vi "log analysis_gps.vi"() -> ()   [LabVIEW 2019] (continued)
0.4458,0.2943,0.5547,0.1143,0.0925,0.0773,0.0983,0.1035,4.8018,0f000001,0*da40ff02\n\t", "INSPVAXA,USB3,0,50.0,FINESTEERING,2107,282792.500,02000000,471d,15824;INS_ALIGNMENT_COMPLETE,INS_RTKFIXED,37.37073031281,126.72411271384,9.9474,22.3000,0.1838,-0.2244,-0.0278,-0.319663676,-2.204085935,299.407243986,0.4460,0.2943,0.5548,0.1143,0.0925,0.0773,0.0983,0.1036,4.8027,0f000001,0*a7b7d02c\n\t", "INSPVAXA,USB3,0,50.0,FINESTEERING,2107,282793.000,02000000,471d,15824;INS_ALIGNMENT_COMPLETE,INS_RTKFIXED,37.37073105512,126.72411141845,9.9418,22.3000,0.2101,-0.2661,-0.0283,-0.304105156,-2.230574791,299.428124027,0.4460,0.2943,0.5548,0.1143,0.0925,0.0773,0.0983,0.1036,4.8027,0f000001,0*32017f41\n\t", "INSPVAXA,USB3,0,48.5,FINESTEERING,2107,282793.500,02000000,471d,15824;INS_ALIGNMENT_COMPLETE,INS_RTKFIXED,37.37073179967,126.72411009506,9.9373,22.3000,0.1839,-0.2284,-0.0293,-0.261169015,-2.357198246,299.469051976,0.4470,0.2945,0.5553,0.1144,0.0927,0.0774,0.0983,0.1036,4.8035,0f000001,0*5198649b\n\t", "INSPVAXA,USB3,0,48.5,FINESTEERING,2107,282794.000,02000000,471d,15824;INS_ALIGNMENT_COMPLETE,INS_RTKFIXED,37.37073258034,126.72410870830,9.9322,22.3000,0.1804,-0.2290,-0.0311,-0.237665421,-2.328772316,299.577236299,0.4470,0.2945,0.5553,0.1144,0.0927,0.0774,0.0983,0.1036,4.8035,0f000001,0*00fdb5a8\n\t", "INSPVAXA,USB3,0,50.0,FINESTEERING,2107,282794.500,02000000,471d,15824;INS_ALIGNMENT_COMPLETE,INS_RTKFIXED,37.37073330075,126.72410740472,9.9287,22.3000,0.1893,-0.2427,-0.0278,-0.202786531,-2.243456476,299.635927133,0.4467,0.2943,0.5552,0.1145,0.0925,0.0773,0.0983,0.1036,4.8037,0f000001,0*5cb0ba92\n\t", "INSPVAXA,USB3,0,50.0,FINESTEERING,2107,282795.000,02000000,471d,15824;INS_ALIGNMENT_COMPLETE,INS_RTKFIXED,37.37073403278,126.72410609803,9.9257,22.3000,0.2016,-0.2553,-0.0322,-0.209242337,-1.998269327,299.675209205,0.4467,0.2943,0.5552,0.1145,0.0925,0.0773,0.0983,0.1036,4.8037,0f000001,0*b5d55d6c\n\t", "INSPVAXA,USB3,0,47.5,FINESTEERING,2107,282795.500,02000000,471d,15824;INS_ALIGNMENT_COMPLETE,INS_RTKFIXED,37.37073477439,126.72410478765,9.9228,22.3000,0.1988,-0.2433,-0.0255,-0.169516872,-1.839910246,299.717118650,0.4468,0.2942,0.5552,0.1144,0.0925,0.0773,0.0984,0.1036,4.8041,0f000001,0*ac4c0833\n\t", "DUALANTENNAHEADINGA,USB3,0,47.5,FINESTEERING,2107,282796.000,02000000,d426,15824;INSUFFICIENT_OBS,NONE,-1.000000000,0.000000000,0.000000000,0.0,0.000000000,0.000000000,\"631T\",16,2,2,2,04,00,20,00*03fa76b0\n\t", "INSPVAXA,USB3,0,49.5,FINESTEERING,2107,282796.500,02000000,471d,15824;INS_ALIGNMENT_COMPLETE,INS_RTKFIXED,37.37073628296,126.72410213089,9.9158,22.3000,0.1865,-0.2481,-0.0343,-0.084207342,-1.811662938,299.819471466,0.4465,0.2941,0.5548,0.1145,0.0924,0.0773,0.0984,0.1036,4.8046,0f000001,0*5f5dfc2c\n\t", "DUALANTENNAHEADINGA,USB3,0,49.5,FINESTEERING,2107,282797.000,02000000,d426,15824;INSUFFICIENT_OBS,NONE,-1.000000000,0.000000000,0.000000000,0.0,0.000000000,0.000000000,\"631T\",11,2,2,2,04,00,20,00*3233b119\n\t", "INSPVAXA,USB3,0,51.0,FINESTEERING,2107,282797.500,02000000,471d,15824;INS_ALIGNMENT_COMPLETE,INS_RTKFIXED,37.37073777614,126.72409945855,9.9099,22.3000,0.1844,-0.2371,-0.0242,-0.262384878,-2.080175298,299.815880388,0.4468,0.2941,0.5547,0.1144,0.0924,0.0773,0.0984,0.1036,4.8050,0f000001,0*8c5fb6f4\n\t", "DUALANTENNAHEADINGA,USB3,0,51.0,FINESTEERING,2107,282798.000,02000000,d426,15824;INSUFFICIENT_OBS,NONE,-1.000000000,0.000000000,0.000000000,0.0,0.000000000,0.000000000,\"631T\",13,2,2,2,04,00,20,00*54bdf9a5\n\t", "DUALANTENNAHEADINGA,USB3,0,48.5,FINESTEERING,2107,282798.500,02000000,d426,15824;INSUFFICIENT_OBS,NONE,-1.000000000,0.000000000,0.000000000,0.0,0.000000000,0.000000000,\"631T\",13,2,2,2,04,00,20,00*f78b4211\n\t", "INSPVAXA,USB3,0,48.5,FINESTEERING,2107,282799.000,02000000,471d,15824;INS_ALIGNMENT_COMPLETE,INS_RTKFIXED,37.37074001096,126.72409550695,9.9018,22.3000,0.1871,-0.2390,-0.0286,-0.222837018,-2.091989069,299.851600763,0.4467,0.2941,0.5546,0.1145,0.0924,0.0773,0.0984,0.1036,4.8055,0f000001,0*154119ed\n\t", "INSPVAXA,USB3,0,48.0,FINESTEERING,2107,282799.500,02000000,471d,15824;INS_ALIGNMENT_COMPLETE,INS_RTKFIXED,37.37074075005,126.72409418540,9.8978,22.3000,0.1813,-0.2293,-0.0193,-0.296668492,-2.062854317,299.895574277,0.4469,0.2941,0.5547,0.1144,0.0924,0.0773,0.0985,0.1036,4.8059,0f000001,0*557f2fd1\n\t", "INSPVAXA,USB3,0,48.0,FINESTEERING,2107,282800.000,02000000,471d,15824;INS_ALIGNMENT_COMPLETE,INS_RTKFIXED,37.37074149494,126.72409286106,9.8944,22.3000,0.1833,-0.2479,-0.0244,-0.375636327,-2.245041894,299.896302450,0.4469,0.2941,0.5547,0.1144,0.0924,0.0773,0.0985,0.1036,4.8059,0f000001,0*618fc424\n\t", "INSPVAXA,USB3,0,50.5,FINESTEERING,2107,282800.500,02000000,471d,15824;INS_ALIGNMENT_COMPLETE,INS_RTKFIXED,37.37074223493,126.72409154227,9.8930,22.3000,0.1953,-0.2548,-0.0229,-0.359173553,-2.315682427,299.885169095,0.4472,0.2942,0.5548,0.1143,0.0924,0.0774,0.0985,0.1036,4.8064,0f000001,0*7582bc0e\n\t", "INSPVAXA,USB3,0,50.5,FINESTEERING,2107,282801.000,02000000,471d,15824;INS_ALIGNMENT_COMPLETE,INS_RTKFIXED,37.37074297365,126.72409022766,9.8906,22.3000,0.1848,-0.2408,-0.0220,-0.434084237,-2.273111027,299.921855092,0.4472,0.2942,0.5548,0.1143,0.0924,0.0774,0.0985,0.1036,4.8064,0f000001,0*0e2f8a3b\n\t", "INSPVAXA,USB3,0,50.5,FINESTEERING,2107,282801.500,02000000,471d,15824;INS_ALIGNMENT_COMPLETE,INS_RTKFIXED,37.37074369952,126.72408891611,9.8878,22.3000,0.1813,-0.2385,-0.0170,-0.522003899,-2.179263420,299.918840889,0.4467,0.2943,0.5547,0.1143,0.0924,0.0773,0.0985,0.1036,4.8071,0f000001,0*ee077a21\n\t", "DUALANTENNAHEADINGA,USB3,0,50.5,FINESTEERING,2107,282802.000,02000000,d426,15824;INSUFFICIENT_OBS,NONE,-1.000000000,0.000000000,0.000000000,0.0,0.000000000,0.000000000,\"631T\",12,2,2,2,04,00,20,00*74fbc462\n\t", "INSPVAXA,USB3,0,47.0,FINESTEERING,2107,282802.500,02000000,471d,15824;INS_ALIGNMENT_COMPLETE,INS_RTKFIXED,37.37074515687,126.72408631213,9.8800,22.3000,0.1804,-0.2401,-0.0128,-0.478381012,-2.174780645,299.958693295,0.4464,0.2943,0.5545,0.1143,0.0924,0.0773,0.0985,0.1036,4.8081,0f000001,0*e501e358\n\t", "DUALANTENNAHEADINGA,USB3,0,47.0,FINESTEERING,2107,282803.000,02000000,d426,15824;INSUFFICIENT_OBS,NONE,-1.000000000,0.000000000,0.000000000,0.0,0.000000000,0.000000000,\"631T\",13,2,2,2,04,00,20,00*accba235\n\t", "DUALANTENNAHEADINGA,USB3,0,45.0,FINESTEERING,2107,282803.500,02000000,d426,15824;INSUFFICIENT_OBS,NONE,-1.000000000,0.000000000,0.000000000,0.0,0.000000000,0.000000000,\"631T\",13,2,2,2,04,00,20,00*b3511e24\n\t", "INSPVAXA,USB3,0,45.0,FINESTEERING,2107,282804.000,02000000,471d,15824;INS_ALIGNMENT_COMPLETE,INS_RTKFIXED,37.37074734035,126.72408240044,9.8696,22.3000,0.1782,-0.2385,-0.0140,-0.685361203,-2.151633306,299.976720233,0.4460,0.2942,0.5542,0.1144,0.0925,0.0773,0.0985,0.1036,4.8092,0f000001,0*10ad259a\n\t", "DUALANTENNAHEADINGA,USB3,0,46.0,FINESTEERING,2107,282804.500,02000000,d426,15824;INSUFFICIENT_OBS,NONE,-1.000000000,0.000000000,0.000000000,0.0,0.000000000,0.000000000,\"631T\",15,2,2,2,04,00,20,00*58397695\n\t", "DUALANTENNAHEADINGA,USB3,0,46.0,FINESTEERING,2107,282805.000,02000000,d426,15824;INSUFFICIENT_OBS,NONE,-1.000000000,0.000000000,0.000000000,0.0,0.000000000,0.000000000,\"631T\",15,2,2,2,04,00,20,00*e2f26315\n\t", "DUALANTENNAHEADINGA,USB3,0,44.5,FINESTEERING,2107,282805.500,02000000,d426,15824;INSUFFICIENT_OBS,NONE,-1.000000000,0.000000000,0.000000000,0.0,0.000000000,0.000000000,\"631T\",15,2,2,2,04,00,20,00*a81239c8\n\t", "DUALANTENNAHEADINGA,USB3,0,44.5,FINESTEERING,2107,282806.000,02000000,d426,15824;INSUFFICIENT_OBS,NONE,-1.000000000,0.000000000,0.000000000,0.0,0.000000000,0.000000000,\"631T\",15,2,2,2,04,00,20,00*c96925fa\n\t", "INSPVAXA,USB3,0,47.5,FINESTEERING,2107,282806.500,02008000,471d,15824;INS_ALIGNMENT_COMPLETE,INS_RTKFIXED,37.37075103198,126.72407599150,9.8611,22.3000,0.1775,-0.2152,-0.0113,-0.726876844,-1.853734910,300.056532649,0.4475,0.2946,0.5549,0.1145,0.0926,0.0774,0.0984,0.1036,4.8109,0f000001,0*336afd29\n\t", "DUALANTENNAHEADINGA,USB3,0,47.5,FINESTEERING,2107,282807.000,02008000,d426,15824;INSUFFICIENT_OBS,NONE,-1.000000000,0.000000000,0.000000000,0.0,0.000000000,0.000000000,\"631T\",15,2,2,2,04,00,20,00*1eefde6e\n\t", "DUALANTENNAHEADINGA,USB3,0,50.5,FINESTEERING,2107,282807.500,02008000,d426,15824;INSUFFICIENT_OBS,NONE,-1.000000000,0.000000000,0.000000000,0.0,0.000000000,0.000000000,\"631T\",15,2,2,2,04,00,20,00*fe8ccb2d\n\t", "INSPVAXA,USB3,0,50.5,FINESTEERING,2107,282808.000,02008000,471d,15824;INS_ALIGNMENT_COMPLETE,INS_RTKFIXED,37.37075325131,126.72407209622,9.8541,22.3000,0.1789,-0.2215,-0.0236,-0.924752960,-1.991766220,300.099829298,0.4478,0.2946,0.5550,0.1144,0.0926,0.0774,0.0984,0.1036,4.8105,0f000001,0*94ebbe09\n\t", "DUALANTENNAHEADINGA,USB3,0,50.0,FINESTEERING,2107,282808.500,02008000,d426,15824;INSUFFICIENT_OBS,NONE,-1.000000000,0.000000000,0.000000000,0.0,0.000000000,0.000000000,\"631T\",14,2,2,2,04,00,20,00*7e4f9fbd\n\t", "DUALANTENNAHEADINGA,USB3,0,50.0,FINESTEERING,2107,282809.000,02008000,d426,15824;INSUFFICIENT_OBS,NONE,-1.000000000,0.000000000,0.000000000,0.0,0.000000000,0.000000000,\"631T\",14,2,2,2,04,00,20,00*c4848a3d\n\t", "DUALANTENNAHEADINGA,USB3,0,48.0,FINESTEERING,2107,282809.500,02008000,d426,15824;INSUFFICIENT_OBS,NONE,-1.000000000,0.000000000,0.000000000,0.0,0.000000000,0.000000000,\"631T\",14,2,2,2,04,00,20,00*568c01e1\n\t", "DUALANTENNAHEADINGA,USB3,0,48.0,FINESTEERING,2107,282810.000,02008000,d426,15824;INSUFFICIENT_OBS,NONE,-1.000000000,0.000000000,0.000000000,0.0,0.000000000,0.000000000,\"631T\",14,2,2,2,04,00,20,00*cb078c5f\n\t", "INSPVAXA,USB3,0,50.0,FINESTEERING,2107,282810.500,02008000,471d,15824;INS_ALIGNMENT_COMPLETE,INS_RTKFIXED,37.37075697026,126.72406559815,9.8397,22.3000,0.1784,-0.2281,-0.0276,-0.963357433,-2.013990950,300.156490692,0.4474,0.2946,0.5550,0.1144,0.0925,0.0774,0.0983,0.1035,4.8086,0f000001,0*76b7c623\n\t", "DUALANTENNAHEADINGA,USB3,0,50.0,FINESTEERING,2107,282811.000,02008000,d426,15824;INSUFFICIENT_OBS,NONE,-1.000000000,0.000000000,0.000000000,0.0,0.000000000,0.000000000,\"631T\",14,2,2,2,04,00,20,00*e3c41203\n\t", "DUALANTENNAHEADINGA,USB3,0,50.0,FINESTEERING,2107,282811.500,02008000,d426,15824;INSUFFICIENT_OBS,NONE,-1.000000000,0.000000000,0.000000000,0.0,0.000000000,0.000000000,\"631T\",15,2,2,2,04,00,20,00*e3358302\n\t", "DUALANTENNAHEADINGA,USB3,0,50.0,FINESTEERING,2107,282812.000,02008000,d426,15824;INSUFFICIENT_OBS,NONE,-1.000000000,0.000000000,0.000000000,0.0,0.000000000,0.000000000,\"631T\",15,2,2,2,04,00,20,00*824e9f30\n\t", "DUALANTENNAHEADINGA,USB3,0,50.0,FINESTEERING,2107,282812.500,02008000,d426,15824;INSUFFICIENT_OBS,NONE,-1.000000000,0.000000000,0.000000000,0.0,0.000000000,0.000000000,\"631T\",14,2,2,2,04,00,20,00*82bf0e31\n\t", "DUALANTENNAHEADINGA,USB3,0,50.0,FINESTEERING,2107,282813.000,02008000,d426,15824;INSUFFICIENT_OBS,NONE,-1.000000000,0.000000000,0.000000000,0.0,0.000000000,0.000000000,\"631T\",12,2,2,2,04,00,20,00*a5a810a2\n\t", "DUALANTENNAHEADINGA,USB3,0,48.0,FINESTEERING,2107,282813.500,02008000,d426,15824;INSUFFICIENT_OBS,NONE,-1.000000000,0.000000000,0.000000000,0.0,0.000000000,0.000000000,\"631T\",11,2,2,2,04,00,20,00*94f61dd7\n\t", "INSPVAXA,USB3,0,48.0,FINESTEERING,2107,282814.000,02008000,471d,15824;INS_ALIGNMENT_COMPLETE,INS_RTKFIXED,37.37076222900,126.72405635034,9.8094,22.3000,0.1883,-0.2144,-0.0181,-0.772460660,-2.046540094,300.011288466,0.4470,0.2944,0.5548,0.1144,0.0924,0.0774,0.0982,0.1035,4.8080,0f000001,0*4e4fcada\n\t", "INSPVAXA,USB3,0,50.0,FINESTEERING,2107,282814.500,02000000,471d,15824;INS_ALIGNMENT_COMPLETE,INS_RTKFIXED,37.37076300208,126.72405500228,9.8062,22.3000,0.1859,-0.2191,-0.0086,-0.683595212,-2.119791281,300.037756065,0.4472,0.2945,0.5552,0.1144,0.0924,0.0774,0.0982,0.1035,4.8084,0f000001,0*aac7df20\n\t", "DUALANTENNAHEADINGA,USB3,0,50.0,FINESTEERING,2107,282815.000,02000000,d426,15824;INSUFFICIENT_OBS,NONE,-1.000000000,0.000000000,0.000000000,0.0,0.000000000,0.000000000,\"631T\",13,2,2,2,04,00,20,00*d37808cc\n\t", "DUALANTENNAHEADINGA,USB3,0,49.0,FINESTEERING,2107,282815.500,02000000,d426,15824;INSUFFICIENT_OBS,NONE,-1.000000000,0.000000000,0.000000000,0.0,0.000000000,0.000000000,\"631T\",12,2,2,2,04,00,20,00*f2d6d5ec\n\t", "DUALANTENNAHEADINGA,USB3,0,49.0,FINESTEERING,2107,282816.000,02000000,d426,15824;INSUFFICIENT_OBS,NONE,-1.000000000,0.000000000,0.000000000,0.0,0.000000000,0.000000000,\"631T\",13,2,2,2,04,00,20,00*444f4986\n\t", "DUALANTENNAHEADINGA,USB3,0,52.0,FINESTEERING,2107,282816.500,02000000,d426,15824;INSUFFICIENT_OBS,NONE,-1.000000000,0.000000000,0.000000000,0.0,0.000000000,0.000000000,\"631T\",12,2,2,2,04,00,20,00*ad6839ee\n\t", "DUALANTENNAHEADINGA,USB3,0,52.0,FINESTEERING,2107,282817.000,02000000,d426,15824;INSUFFICIENT_OBS,NONE,-1.000000000,0.000000000,0.000000000,0.0,0.000000000,0.000000000,\"631T\",14,2,2,2,04,00,20,00*8a7f277d\n\t", "DUALANTENNAHEADINGA,USB3,0,47.0,FINESTEERING,2107,282817.500,02000000,d426,15824;INSUFFICIENT_OBS,NONE,-1.000000000,0.000000000,0.000000000,0.0,0.000000000,0.000000000,\"631T\",13,2,2,2,04,00,20,00*e8ab143d\n\t", "DUALANTENNAHEADINGA,USB3,0,47.0,FINESTEERING,2107,282818.000,02000000,d426,15824;INSUFFICIENT_OBS,NONE,-1.000000000,0.000000000,0.000000000,0.0,0.000000000,0.000000000,\"631T\",11,2,2,2,04,00,20,00*49573191\n\t", "DUALANTENNAHEADINGA,USB3,0,45.5,FINESTEERING,2107,282818.500,02000000,d426,15824;INSUFFICIENT_OBS,NONE,-1.000000000,0.000000000,0.000000000,0.0,0.000000000,0.000000000,\"631T\",11,2,2,2,04,00,20,00*03b76b4c\n\t", "DUALANTENNAHEADINGA,USB3,0,45.5,FINESTEERING,2107,282819.000,02000000,d426,15824;INSUFFICIENT_OBS,NONE,-1.000000000,0.000000000,0.000000000,0.0,0.000000000,0.000000000,\"631T\",12,2,2,2,04,00,20,00*1a2af865\n\t", "DUALANTENNAHEADINGA,USB3,0,50.5,FINESTEERING,2107,282819.500,02000000,d426,15824;INSUFFICIENT_OBS,NONE,-1.000000000,0.000000000,0.000000000,0.0,0.000000000,0.000000000,\"631T\",13,2,2,2,04,00,20,00*e522c036\n\t", "DUALANTENNAHEADINGA,USB3,0,50.5,FINESTEERING,2107,282820.000,02000000,d426,15824;INSUFFICIENT_OBS,NONE,-1.000000000,0.000000000,0.000000000,0.0,0.000000000,0.000000000,\"631T\",14,2,2,2,04,00,20,00*1723a46a\n\t", "DUALANTENNAHEADINGA,USB3,0,50.5,FINESTEERING,2107,282820.500,02008000,d426,15824;INSUFFICIENT_OBS,NONE,-1.000000000,0.000000000,0.000000000,0.0,0.000000000,0.000000000,\"631T\",14,2,2,2,04,00,20,00*d6a33192\n\t", "DUALANTENNAHEADINGA,USB3,0,50.5,FINESTEERING,2107,282821.000,02008000,d426,15824;INSUFFICIENT_OBS,NONE,-1.000000000,0.000000000,0.000000000,0.0,0.000000000,0.000000000,\"631T\",16,2,2,2,04,00,20,00*18dc22e3\n\t", "DUALANTENNAHEADINGA,USB3,0,50.0,FINESTEERING,2107,282822.000,02008000,d426,15824;INSUFFICIENT_OBS,NONE,-1.000000000,0.000000000,0.000000000,0.0,0.000000000,0.000000000,\"631T\",16,2,2,2,04,00,20,00*fbcec944\n\t", "DUALANTENNAHEADINGA,USB3,0,49.0,FINESTEERING,2107,282822.500,02008000,d426,15824;INSUFFICIENT_OBS,NONE,-1.000000000,0.000000000,0.000000000,0.0,0.000000000,0.000000000,\"631T\",15,2,2,2,04,00,20,00*aed41295\n\t", "DUALANTENNAHEADINGA,USB3,0,49.0,FINESTEERING,2107,282823.000,02008000,d426,15824;INSUFFICIENT_OBS,NONE,-1.000000000,0.000000000,0.000000000,0.0,0.000000000,0.000000000,\"631T\",15,2,2,2,04,00,20,00*141f0715\n\t", "DUALANTENNAHEADINGA,USB3,0,45.5,FINESTEERING,2107,282823.500,02008000,d426,15824;INSUFFICIENT_OBS,NONE,-1.000000000,0.000000000,0.000000000,0.0,0.000000000,0.000000000,\"631T\",14,2,2,2,04,00,20,00*9f3295ab\n\t", "DUALANTENNAHEADINGA,USB3,0,45.5,FINESTEERING,2107,282824.000,02008000,d426,15824;INSUFFICIENT_OBS,NONE,-1.000000000,0.000000000,0.000000000,0.0,0.000000000,0.000000000,\"631T\",12,2,2,2,04,00,20,00*0f8497af\n\t", "DUALANTENNAHEADINGA,USB3,0,50.5,FINESTEERING,2107,282824.500,02000000,d426,15824;INSUFFICIENT_OBS,NONE,-1.000000000,0.000000000,0.000000000,0.0,0.000000000,0.000000000,\"631T\",12,2,2,2,04,00,20,00*31fdab05\n\t", "DUALANTENNAHEADINGA,USB3,0,50.5,FINESTEERING,2107,282825.000,02000000,d426,15824;INSUFFICIENT_OBS,NONE,-1.000000000,0.000000000,0.000000000,0.0,0.000000000,0.000000000,\"631T\",14,2,2,2,04,00,20,00*16eab596\n\t", "DUALANTENNAHEADINGA,USB3,0,49.5,FINESTEERING,2107,282825.500,02000000,d426,15824;INSUFFICIENT_OBS,NONE,-1.000000000,0.000000000,0.000000000,0.0,0.000000000,0.000000000,\"631T\",16,2,2,2,04,00,20,00*9412ee1f\n\t", "DUALANTENNAHEADINGA,USB3,0,49.5,FINESTEERING,2107,282826.000,02000000,d426,15824;INSUFFICIENT_OBS,NONE,-1.000000000,0.000000000,0.000000000,0.0,0.000000000,0.000000000,\"631T\",15,2,2,2,04,00,20,00*563f7484\n\t", "DUALANTENNAHEADINGA,USB3,0,48.5,FINESTEERING,2107,282827.000,02000000,d426,15824;INSUFFICIENT_OBS,NONE,-1.000000000,0.000000000,0.000000000,0.0,0.000000000,0.000000000,\"631T\",15,2,2,2,04,00,20,00*5fa3a6f9\n\t", "DUALANTENNAHEADINGA,USB3,0,47.0,FINESTEERING,2107,282827.500,02000000,d426,15824;INSUFFICIENT_OBS,NONE,-1.000000000,0.000000000,0.000000000,0.0,0.000000000,0.000000000,\"631T\",14,2,2,2,04,00,20,00*78434fab\n\t", "DUALANTENNAHEADINGA,USB3,0,47.0,FINESTEERING,2107,282828.000,02000000,d426,15824;INSUFFICIENT_OBS,NONE,-1.000000000,0.000000000,0.000000000,0.0,0.000000000,0.000000000,\"631T\",14,2,2,2,04,00,20,00*ad0b6cf6\n\t", "DUALANTENNAHEADINGA,USB3,0,50.0,FINESTEERING,2107,282828.500,02000000,d426,15824;INSUFFICIENT_OBS,NONE,-1.000000000,0.000000000,0.000000000,0.0,0.000000000,0.000000000,\"631T\",14,2,2,2,04,00,20,00*4d6879b5\n\t", "DUALANTENNAHEADINGA,USB3,0,50.0,FINESTEERING,2107,282829.000,02000000,d426,15824;INSUFFICIENT_OBS,NONE,-1.000000000,0.000000000,0.000000000,0.0,0.000000000,0.000000000,\"631T\",14,2,2,2,04,00,20,00*f7a36c35\n\t", "DUALANTENNAHEADINGA,USB3,0,51.0,FINESTEERING,2107,282829.500,02000000,d426,15824;INSUFFICIENT_OBS,NONE,-1.000000000,0.000000000,0.000000000,0.0,0.000000000,0.000000000,\"631T\",15,2,2,2,04,00,20,00*93162b90\n\t", "INSPVAXA,USB3,0,51.0,FINESTEERING,2107,282830.050,02000000,471d,15824;INS_ALIGNMENT_COMPLETE,INS_RTKFIXED,37.37078622103,126.72401367008,9.6748,22.3000,0.1678,-0.2481,-0.0115,-0.997229556,-1.986004946,301.087266314,0.4437,0.2943,0.5539,0.1140,0.0924,0.0773,0.0983,0.1033,4.8231,0f000001,0*4fbfc59a\n\t", "DUALANTENNAHEADINGA,USB3,0,51.5,FINESTEERING,2107,282831.000,02000000,d426,15824;INSUFFICIENT_OBS,NONE,-1.000000000,0.000000000,0.000000000,0.0,0.000000000,0.000000000,\"631T\",14,2,2,2,04,00,20,00*e1ddc463\n\t", "INSPVAXA,USB3,0,50.0,FINESTEERING,2107,282831.550,02000000,471d,15824;INS_ALIGNMENT_COMPLETE,INS_RTKFIXED,37.37078850340,126.72400981553,9.6631,22.3000,0.1496,-0.2201,-0.0118,-1.048727398,-2.216278260,301.282066784,0.4433,0.2942,0.5538,0.1139,0.0924,0.0773,0.0983,0.1033,4.8246,0f000001,0*7f01e368\n\t", "DUALANTENNAHEADINGA,USB3,0,47.0,FINESTEERING,2107,282832.500,02000000,d426,15824;INSUFFICIENT_OBS,NONE,-1.000000000,0.000000000,0.000000000,0.0,0.000000000,0.000000000,\"631T\",16,2,2,2,04,00,20,00*f25cead2\n\t", "INSPVAXA,USB3,0,47.0,FINESTEERING,2107,282833.050,02000000,471d,15824;INS_ALIGNMENT_COMPLETE,INS_RTKFIXED,37.37079076592,126.72400610442,9.6518,22.3000,0.1650,-0.2502,-0.0160,-0.860770994,-2.117713519,301.563204490,0.4421,0.2941,0.5532,0.1138,0.0924,0.0773,0.0983,0.1033,4.8276,0f000001,0*c29dada0\n\t", "DUALANTENNAHEADINGA,USB3,0,50.5,FINESTEERING,2107,282833.500,02000000,d426,15824;INSUFFICIENT_OBS,NONE,-1.000000000,0.000000000,0.000000000,0.0,0.000000000,0.000000000,\"631T\",14,2,2,2,04,00,20,00*893a0a2c\n\t", "DUALANTENNAHEADINGA,USB3,0,47.5,FINESTEERING,2107,282834.500,02000000,d426,15824;INSUFFICIENT_OBS,NONE,-1.000000000,0.000000000,0.000000000,0.0,0.000000000,0.000000000,\"631T\",16,2,2,2,04,00,20,00*10871089\n\t", "INSPVAXA,USB3,0,47.5,FINESTEERING,2107,282835.050,02000000,471d,15824;INS_ALIGNMENT_COMPLETE,INS_RTKFIXED,37.37079382962,126.72400108801,9.6374,22.3000,0.1569,-0.2281,-0.0111,-0.999674572,-2.085636983,301.443482379,0.4416,0.2941,0.5526,0.1138,0.0924,0.0773,0.0983,0.1033,4.8306,0f000001,0*021b0f77\n\t", "INSPVAXA,USB3,0,49.0,FINESTEERING,2107,282835.550,02000000,471d,15824;INS_ALIGNMENT_COMPLETE,INS_RTKFIXED,37.37079461184,126.72399982045,9.6347,22.3000,0.1482,-0.2050,-0.0185,-0.996168603,-2.046587812,301.390130143,0.4416,0.2941,0.5526,0.1138,0.0924,0.0773,0.0983,0.1033,4.8306,0f000001,0*e466e7db\n\t", "INSPVAXA,USB3,0,49.5,FINESTEERING,2107,282836.550,02000000,471d,15824;INS_ALIGNMENT_COMPLETE,INS_RTKFIXED,37.37079614762,126.72399733501,9.6280,22.3000,0.1600,-0.2167,-0.0303,-0.871497210,-2.188105469,301.034385182,0.4418,0.2941,0.5524,0.1139,0.0924,0.0773,0.0983,0.1033,4.8319,0f000001,0*58ef0c84\n\t", "INSPVAXA,USB3,0,48.5,FINESTEERING,2107,282837.050,02000000,471d,15824;INS_ALIGNMENT_COMPLETE,INS_RTKFIXED,37.37079689035,126.72399612134,9.6249,22.3000,0.1550,-0.2065,-0.0179,-0.785589438,-2.162266254,300.814007904,0.4425,0.2941,0.5525,0.1140,0.0924,0.0773,0.0983,0.1033,4.8330,0f000001,0*63c71cff\n\t", "INSPVAXA,USB3,0,48.5,FINESTEERING,2107,282837.550,02000000,471d,15824;INS_ALIGNMENT_COMPLETE,INS_RTKFIXED,37.37079762799,126.72399488402,9.6202,22.3000,0.1524,-0.1993,-0.0171,-0.713862007,-2.052581994,300.562898535,0.4425,0.2941,0.5525,0.1140,0.0924,0.0773,0.0983,0.1033,4.8330,0f000001,0*d3644a20\n\t", "INSPVAXA,USB3,0,49.5,FINESTEERING,2107,282838.550,02000000,471d,15824;INS_ALIGNMENT_COMPLETE,INS_RTKFIXED,37.37079907064,126.72399237464,9.6125,22.3000,0.1577,-0.2192,-0.0140,-0.837165227,-1.670419356,300.018600301,0.4429,0.2941,0.5524,0.1143,0.0924,0.0773,0.0982,0.1033,4.8338,0f000001,0*758de772\n\t", "INSPVAXA,USB3,0,49.5,FINESTEERING,2107,282839.050,02000000,471d,15824;INS_ALIGNMENT_COMPLETE,INS_RTKFIXED,37.37079978171,126.72399113225,9.6082,22.3000,0.1499,-0.2017,-0.0243,-0.847366438,-1.584995837,299.787057757,0.4435,0.2941,0.5523,0.1144,0.0925,0.0773,0.0982,0.1033,4.8337,0f000001,0*2af0ce7f\n\t", "INSPVAXA,USB3,0,51.0,FINESTEERING,2107,282839.550,02000000,471d,15824;INS_ALIGNMENT_COMPLETE,INS_RTKFIXED,37.37080052394,126.72398985335,9.6041,22.3000,0.1541,-0.2085,-0.0197,-0.657538582,-1.555388056,299.628697476,0.4435,0.2941,0.5523,0.1144,0.0925,0.0773,0.0982,0.1033,4.8337,0f000001,0*e249b229\n\t", "INSPVAXA,USB3,0,50.5,FINESTEERING,2107,282840.550,02000000,471d,15824;INS_ALIGNMENT_COMPLETE,INS_RTKFIXED,37.37080198086,126.72398726607,9.5945,22.3000,0.1415,-0.2075,-0.0192,-0.681588994,-1.930393004,299.482671572,0.4442,0.2942,0.5523,0.1142,0.0924,0.0773,0.0982,0.1033,4.8325,0f000001,0*f7245bcc\n\t", "INSPVAXA,USB3,0,50.5,FINESTEERING,2107,282841.050,02000000,471d,15824;INS_ALIGNMENT_COMPLETE,INS_RTKFIXED,37.37080269801,126.72398599204,9.5896,22.3000,0.1407,-0.1883,-0.0149,-0.746862353,-2.032009103,299.450305657,0.4442,0.2942,0.5522,0.1141,0.0924,0.0773,0.0982,0.1032,4.8310,0f000001,0*0739b113\n\t", "INSPVAXA,USB3,0,47.0,FINESTEERING,2107,282841.550,02000000,471d,15824;INS_ALIGNMENT_COMPLETE,INS_RTKFIXED,37.37080343630,126.72398465654,9.5859,22.3000,0.1441,-0.2016,-0.0158,-0.831480071,-2.195246795,299.385489807,0.4442,0.2942,0.5522,0.1141,0.0924,0.0773,0.0982,0.1032,4.8310,0f000001,0*a0ec8594\n\t", "INSPVAXA,USB3,0,46.5,FINESTEERING,2107,282842.050,02000000,471d,15824;INS_ALIGNMENT_COMPLETE,INS_RTKFIXED,37.37080417345,126.72398334114,9.5820,22.3000,0.1511,-0.2042,-0.0206,-0.794633403,-2.254519225,299.313785412,0.4438,0.2942,0.5520,0.1137,0.0924,0.0772,0.0982,0.1032,4.8295,0f000001,0*390828f0\n\t", "INSPVAXA,USB3,0,46.5,FINESTEERING,2107,282842.550,02000000,471d,15824;INS_ALIGNMENT_COMPLETE,INS_RTKFIXED,37.37080492291,126.72398204575,9.5781,22.3000,0.1466,-0.2045,-0.0217,-0.587846537,-2.261082521,299.368921912,0.4438,0.2942,0.5520,0.1137,0.0924,0.0772,0.0982,0.1032,4.8295,0f000001,0*9ddbd7c7\n\t", "INSPVAXA,USB3,0,46.5,FINESTEERING,2107,282843.050,02000000,471d,15824;INS_ALIGNMENT_COMPLETE,INS_RTKFIXED,37.37080566870,126.72398074821,9.5741,22.3000,0.1339,-0.1915,-0.0133,-0.480026925,-2.203118399,299.401112268,0.4434,0.2940,0.5520,0.1139,0.0924,0.0772,0.0981,0.1031,4.8288,0f000001,0*1d5f5b91\n\t", "INSPVAXA,USB3,0,48.0,FINESTEERING,2107,282843.550,02000000,471d,15824;INS_ALIGNMENT_COMPLETE,INS_RTKFIXED,37.37080641021,126.72397942469,9.5707,22.3000,0.1423,-0.2057,-0.0134,-0.517073533,-2.121653000,299.405019145,0.4434,0.2940,0.5520,0.1139,0.0924,0.0772,0.0981,0.1031,4.8288,0f000001,0*aad3db2c\n\t", "DUALANTENNAHEADINGA,USB3,0,46.5,FINESTEERING,2107,282844.500,02000000,d426,15824;INSUFFICIENT_OBS,NONE,-1.000000000,0.000000000,0.000000000,0.0,0.000000000,0.000000000,\"631T\",14,2,2,2,04,00,20,00*91c9d553\n\t", "INSPVAXA,USB3,0,46.5,FINESTEERING,2107,282845.050,02000000,471d,15824;INS_ALIGNMENT_COMPLETE,INS_RTKFIXED,37.37080866547,126.72397546111,9.5573,22.3000,0.1531,-0.2061,-0.0195,-0.434360785,-2.083992757,299.534678946,0.4435,0.2939,0.5519,0.1137,0.0924,0.0772,0.0981,0.1031,4.8277,0f000001,0*84ceebbb\n\t", "INSPVAXA,USB3,0,48.5,FINESTEERING,2107,282845.550,02000000,471d,15824;INS_ALIGNMENT_COMPLETE,INS_RTKFIXED,37.37080941702,126.72397412031,9.5548,22.3000,0.1626,-0.2203,-0.0192,-0.594420667,-2.098021967,299.551674256,0.4435,0.2939,0.5519,0.1137,0.0924,0.0772,0.0981,0.1031,4.8277,0f000001,0*c2a985dc\n\t", "INSPVAXA,USB3,0,47.5,FINESTEERING,2107,282846.050,02000000,471d,15824;INS_ALIGNMENT_COMPLETE,INS_RTKFIXED,37.37081017945,126.72397278683,9.5521,22.3000,0.1549,-0.2109,-0.0140,-0.604914668,-2.152808656,299.610978470,0.4432,0.2939,0.5518,0.1137,0.0924,0.0772,0.0981,0.1031,4.8275,0f000001,0*a6608b47\n\t", "INSPVAXA,USB3,0,47.5,FINESTEERING,2107,282846.550,02000000,471d,15824;INS_ALIGNMENT_COMPLETE,INS_RTKFIXED,37.37081095004,126.72397139929,9.5473,22.3000,0.1385,-0.1894,-0.0029,-0.694805946,-2.128009753,299.688157025,0.4432,0.2939,0.5518,0.1137,0.0924,0.0772,0.0981,0.1031,4.8275,0f000001,0*5d110ef8\n\t", "INSPVAXA,USB3,0,44.5,FINESTEERING,2107,282847.050,02000000,471d,15824;INS_ALIGNMENT_COMPLETE,INS_RTKFIXED,37.37081171742,126.72397003068,9.5427,22.3000,0.1573,-0.2192,-0.0020,-0.777578191,-2.007727791,299.761533607,0.4435,0.2940,0.5521,0.1137,0.0924,0.0772,0.0981,0.1031,4.8277,0f000001,0*78548d8e\n\t", "INSPVAXA,USB3,0,44.5,FINESTEERING,2107,282847.550,02000000,471d,15824;INS_ALIGNMENT_COMPLETE,INS_RTKFIXED,37.37081244961,126.72396875131,9.5405,22.3000,0.1641,-0.2218,-0.0106,-0.802151330,-1.920952187,299.784241204,0.4435,0.2940,0.5521,0.1137,0.0924,0.0772,0.0981,0.1031,4.8277,0f000001,0*07f3c654\n\t", "INSPVAXA,USB3,0,44.5,FINESTEERING,2107,282848.050,02000000,471d,15824;INS_ALIGNMENT_COMPLETE,INS_RTKFIXED,37.37081323454,126.72396738661,9.5387,22.3000,0.1349,-0.1756,0.0025,-0.775318763,-1.846543645,299.874004513,0.4431,0.2940,0.5522,0.1139,0.0924,0.0772,0.0981,0.1031,4.8282,0f000001,0*cf4a726c\n\t", "INSPVAXA,USB3,0,45.0,FINESTEERING,2107,282848.550,02000000,471d,15824;INS_ALIGNMENT_COMPLETE,INS_RTKFIXED,37.37081402726,126.72396600462,9.5360,22.3000,0.1572,-0.2154,0.0012,-0.746342979,-1.873663068,299.943587251,0.4431,0.2940,0.5522,0.1139,0.0924,0.0772,0.0981,0.1031,4.8282,0f000001,0*b8902195\n\t", "INSPVAXA,USB3,0,44.5,FINESTEERING,2107,282849.050,02000000,471d,15824;INS_ALIGNMENT_COMPLETE,INS_RTKFIXED,37.37081477161,126.72396469278,9.5343,22.3000,0.1752,-0.2340,-0.0030,-0.967406994,-1.848268930,299.977215039,0.4433,0.2941,0.5523,0.1136,0.0924,0.0772,0.0981,0.1031,4.8286,0f000001,0*2493a191\n\t", "INSPVAXA,USB3,0,44.5,FINESTEERING,2107,282849.550,02000000,471d,15824;INS_ALIGNMENT_COMPLETE,INS_RTKFIXED,37.37081552203,126.72396337229,9.5340,22.3000,0.1625,-0.2097,0.0040,-0.944405978,-1.796098220,300.013826004,0.4433,0.2941,0.5523,0.1136,0.0924,0.0772,0.0981,0.1031,4.8286,0f000001,0*6a619609\n\t", "INSPVAXA,USB3,0,44.5,FINESTEERING,2107,282850.050,02000000,471d,15824;INS_ALIGNMENT_COMPLETE,INS_RTKFIXED,37.37081628430,126.72396202369,9.5336,22.3000,0.1377,-0.1761,0.0033,-0.977356975,-1.557691035,300.050326514,0.4426,0.2941,0.5523,0.1138,0.0925,0.0772,0.0981,0.1030,4.8295,0f000001,0*a61f27a1\n\t", "INSPVAXA,USB3,0,47.5,FINESTEERING,2107,282850.550,02000000,471d,15824;INS_ALIGNMENT_COMPLETE,INS_RTKFIXED,37.37081707791,126.72396063586,9.5326,22.3000,0.1576,-0.1997,0.0014,-0.911286398,-1.407612709,300.113222709,0.4426,0.2941,0.5523,0.1138,0.0925,0.0772,0.0981,0.1030,4.8295,0f000001,0*c59ed98f\n\t", "INSPVAXA,USB3,0,47.5,FINESTEERING,2107,282851.050,02000000,471d,15824;INS_ALIGNMENT_COMPLETE,INS_RTKFIXED,37.37081784915,126.72395932045,9.5307,22.3000,0.1604,-0.2227,0.0007,-0.811075284,-1.430938970,300.158787074,0.4420,0.2942,0.5520,0.1135,0.0924,0.0772,0.0981,0.1030,4.8299,0f000001,0*3724944b\n\t", "INSPVAXA,USB3,0,50.0,FINESTEERING,2107,282851.550,02000000,471d,15824;INS_ALIGNMENT_COMPLETE,INS_RTKFIXED,37.37081861345,126.72395800267,9.5292,22.3000,0.1561,-0.2014,0.0080,-0.732820805,-1.409359332,300.160206583,0.4420,0.2942,0.5520,0.1135,0.0924,0.0772,0.0981,0.1030,4.8299,0f000001,0*b9091ec1\n\t", "INSPVAXA,USB3,0,41.5,FINESTEERING,2107,282852.050,02000000,471d,15824;INS_ALIGNMENT_COMPLETE,INS_RTKFIXED,37.37081939468,126.72395663812,9.5281,22.3000,0.1575,-0.2070,-0.0013,-0.818147595,-1.685386594,300.178906783,0.4415,0.2941,0.5518,0.1134,0.0924,0.0772,0.0981,0.1030,4.8305,0f000001,0*5aa17ff6\n\t", "INSPVAXA,USB3,0,47.5,FINESTEERING,2107,282855.050,02000000,471d,15824;INS_ALIGNMENT_COMPLETE,INS_RTKFIXED,37.37082400176,126.72394869235,9.5093,22.3000,0.1580,-0.2046,-0.0114,-0.756987003,-2.231320148,300.245266772,0.4400,0.2940,0.5516,0.1134,0.0924,0.0772,0.0981,0.1030,4.8343,0f000001,0*a1d38784\n\t", "INSPVAXA,USB3,0,48.0,FINESTEERING,2107,282855.550,02000000,471d,15824;INS_ALIGNMENT_COMPLETE,INS_RTKFIXED,37.37082475865,126.72394738015,9.5053,22.3000,0.1620,-0.1986,-0.0100,-0.702343381,-2.122687121,300.199626754,0.4400,0.2940,0.5516,0.1134,0.0924,0.0772,0.0981,0.1030,4.8343,0f000001,0*af41ec57\n\t", "INSPVAXA,USB3,0,46.5,FINESTEERING,2107,282856.050,02008000,471d,15824;INS_ALIGNMENT_COMPLETE,INS_RTKFIXED,37.37082551882,126.72394606788,9.5018,22.3000,0.1724,-0.2105,-0.0168,-0.698987302,-1.986256005,300.182498357,0.4393,0.2939,0.5514,0.1133,0.0924,0.0772,0.0981,0.1030,4.8357,0f000001,0*2de35edc\n\t", "INSPVAXA,USB3,0,51.5,FINESTEERING,2107,282857.550,02008000,471d,15824;INS_ALIGNMENT_COMPLETE,INS_RTKFIXED,37.37082778753,126.72394219163,9.4923,22.3000,0.1642,-0.2009,-0.0151,-0.455107252,-1.810033780,299.964612436,0.4399,0.2940,0.5516,0.1134,0.0924,0.0772,0.0981,0.1030,4.8372,0f000001,0*479a7bb4\n\t", "INSPVAXA,USB3,0,49.5,FINESTEERING,2107,282858.050,02008000,471d,15824;INS_ALIGNMENT_COMPLETE,INS_RTKFIXED,37.37082854374,126.72394089011,9.4899,22.3000,0.1736,-0.2113,-0.0068,-0.453429457,-1.745153830,299.927988813,0.4398,0.2940,0.5516,0.1134,0.0924,0.0772,0.0981,0.1030,4.8386,0f000001,0*54a30be2\n\t", "INSPVAXA,USB3,0,48.5,FINESTEERING,2107,282859.550,02008000,471d,15824;INS_ALIGNMENT_COMPLETE,INS_RTKFIXED,37.37083079066,126.72393699083,9.4791,22.3000,0.1717,-0.2000,-0.0121,-0.342154854,-1.629050926,299.761505256,0.4409,0.2941,0.5521,0.1136,0.0924,0.0772,0.0981,0.1030,4.8401,0f000001,0*7242c930\n\t", "INSPVAXA,USB3,0,48.5,FINESTEERING,2107,282860.050,02008000,471d,15824;INS_ALIGNMENT_COMPLETE,INS_RTKFIXED,37.37083153175,126.72393569297,9.4766,22.3000,0.1682,-0.1931,-0.0033,-0.310568947,-1.805942662,299.681002094,0.4411,0.2941,0.5523,0.1135,0.0924,0.0772,0.0981,0.1030,4.8414,0f000001,0*16d456af\n\t", "INSPVAXA,USB3,0,51.0,FINESTEERING,2107,282860.550,02000000,471d,15824;INS_ALIGNMENT_COMPLETE,INS_RTKFIXED,37.37083229529,126.72393437190,9.4736,22.3000,0.1681,-0.2003,0.0025,-0.225394302,-1.975265163,299.646950177,0.4411,0.2941,0.5523,0.1135,0.0924,0.0772,0.0981,0.1030,4.8414,0f000001,0*68c0c475\n\t", "INSPVAXA,USB3,0,49.5,FINESTEERING,2107,282861.550,02000000,471d,15824;INS_ALIGNMENT_COMPLETE,INS_RTKFIXED,37.37083383059,126.72393172727,9.4648,22.3000,0.1776,-0.2087,-0.0050,-0.195119204,-2.063452945,299.576804246,0.4408,0.2940,0.5521,0.1134,0.0924,0.0772,0.0981,0.1030,4.8426,0f000001,0*61c3be3c\n\t", "INSPVAXA,USB3,0,43.5,FINESTEERING,2107,282863.050,02000000,471d,15824;INS_ALIGNMENT_COMPLETE,INS_RTKFIXED,37.37083613532,126.72392778169,9.4521,22.3000,0.1728,-0.2101,-0.0119,-0.074623458,-1.995146036,299.426549477,0.4414,0.2940,0.5522,0.1135,0.0924,0.0772,0.0981,0.1030,4.8451,0f000001,0*1428b524\n\t", "INSPVAXA,USB3,0,51.5,FINESTEERING,2107,282866.550,02000000,471d,15824;INS_ALIGNMENT_COMPLETE,INS_RTKFIXED,37.37084144931,126.72391854288,9.4238,22.3000,0.1586,-0.1939,-0.0075,-0.000254507,-1.973115927,299.207530443,0.4415,0.2941,0.5523,0.1135,0.0924,0.0772,0.0981,0.1030,4.8486,0f000001,0*7419bcbe\n\t", "INSPVAXA,USB3,0,49.0,FINESTEERING,2107,282869.550,02000000,471d,15824;INS_ALIGNMENT_COMPLETE,INS_RTKFIXED,37.37084591641,126.72391064457,9.4025,22.3000,0.1631,-0.2087,-0.0091,0.094919053,-1.740347092,299.016545288,0.4419,0.2942,0.5525,0.1136,0.0924,0.0772,0.0981,0.1030,4.8515,0f000001,0*b4375d21\n\t", "INSPVAXA,USB3,0,47.0,FINESTEERING,2107,282885.600,02008000,471d,15824;INS_ALIGNMENT_COMPLETE,INS_RTKFIXED,37.37087024505,126.72386724376,9.2438,22.3000,0.1935,-0.2367,-0.0200,-0.555619573,-2.649892401,299.303581082,0.4421,0.2945,0.5549,0.1137,0.0925,0.0774,0.0981,0.1030,4.8706,0f000001,0*97a1aad7\n\t", "INSPVAXA,USB3,0,44.0,FINESTEERING,2107,282888.100,02000000,471d,15824;INS_ALIGNMENT_COMPLETE,INS_RTKFIXED,37.37087398802,126.72386055207,9.2130,22.3000,0.1784,-0.2231,-0.0172,-0.474670007,-2.406033288,299.373176614,0.4412,0.2944,0.5546,0.1136,0.0925,0.0773,0.0980,0.1030,4.8749,0f000001,0*64b8e8ef\n\t", "INSPVAXA,USB3,0,48.5,FINESTEERING,2107,282895.100,02000000,471d,15824;INS_ALIGNMENT_COMPLETE,INS_RTKFIXED,37.37088448799,126.72384205034,9.1438,22.3000,0.1933,-0.2424,-0.0028,-0.201390353,-2.093342605,299.449772344,0.4447,0.2945,0.5555,0.1140,0.0925,0.0774,0.0980,0.1030,4.8838,0f000001,0*927e2c09\n\t", "INSPVAXA,USB3,0,48.5,FINESTEERING,2107,282895.600,02000000,471d,15824;INS_ALIGNMENT_COMPLETE,INS_RTKFIXED,37.37088525085,126.72384071933,9.1382,22.3000,0.1891,-0.2249,-0.0147,-0.298436977,-2.149365506,299.431607145,0.4447,0.2945,0.5555,0.1140,0.0925,0.0774,0.0980,0.1030,4.8838,0f000001,0*8cb89ae5\n\t", "INSPVAXA,USB3,0,50.0,FINESTEERING,2107,282896.100,02000000,471d,15824;INS_ALIGNMENT_COMPLETE,INS_RTKFIXED,37.37088602098,126.72383942643,9.1321,22.3000,0.1872,-0.2208,-0.0098,-0.216671820,-2.100330729,299.377504290,0.4449,0.2945,0.5555,0.1140,0.0925,0.0774,0.0980,0.1030,4.8845,0f000001,0*ef0b4927\n\t", "INSPVAXA,USB3,0,50.0,FINESTEERING,2107,282896.600,02000000,471d,15824;INS_ALIGNMENT_COMPLETE,INS_RTKFIXED,37.37088675072,126.72383814980,9.1274,22.3000,0.1877,-0.2084,-0.0156,-0.228208842,-2.023017787,299.331781816,0.4449,0.2945,0.5555,0.1140,0.0925,0.0774,0.0980,0.1030,4.8845,0f000001,0*c594017f\n\t", "INSPVAXA,USB3,0,50.5,FINESTEERING,2107,282897.100,02000000,471d,15824;INS_ALIGNMENT_COMPLETE,INS_RTKFIXED,37.37088750252,126.72383685308,9.1243,22.3000,0.1876,-0.2107,-0.0114,-0.201079382,-2.183646945,299.196189709,0.4447,0.2943,0.5554,0.1139,0.0925,0.0774,0.0980,0.1030,4.8850,0f000001,0*259ceb0e\n\t", "INSPVAXA,USB3,0,50.5,FINESTEERING,2107,282897.600,02000000,471d,15824;INS_ALIGNMENT_COMPLETE,INS_RTKFIXED,37.37088825874,126.72383552871,9.1219,22.3000,0.1981,-0.2184,-0.0197,-0.162513691,-2.197478943,299.137776460,0.4447,0.2943,0.5554,0.1139,0.0925,0.0774,0.0980,0.1030,4.8850,0f000001,0*0c5abc39\n\t", "INSPVAXA,USB3,0,49.5,FINESTEERING,2107,282898.100,02000000,471d,15824;INS_ALIGNMENT_COMPLETE,INS_RTKFIXED,37.37088900648,126.72383424276,9.1196,22.3000,0.2094,-0.2215,-0.0185,-0.097507181,-2.148657540,298.990101476,0.4444,0.2942,0.5550,0.1138,0.0925,0.0774,0.0981,0.1030,4.8854,0f000001,0*b8bcb2e5\n\t", "INSPVAXA,USB3,0,44.5,FINESTEERING,2107,282901.100,02000000,471d,15824;INS_ALIGNMENT_COMPLETE,INS_RTKFIXED,37.37089345276,126.72382632257,9.1013,22.3000,0.2073,-0.2174,-0.0049,0.127947696,-2.049748095,298.428012229,0.4429,0.2942,0.5542,0.1136,0.0924,0.0773,0.0981,0.1029,4.8869,0f000001,0*2739f994\n\t", "INSPVAXA,USB3,0,44.5,FINESTEERING,2107,282901.600,02000000,471d,15824;INS_ALIGNMENT_COMPLETE,INS_RTKFIXED,37.37089417130,126.72382498099,9.0979,22.3000,0.2123,-0.2139,-0.0112,0.110382768,-2.113702114,298.389030042,0.4429,0.2942,0.5542,0.1136,0.0924,0.0773,0.0981,0.1029,4.8869,0f000001,0*7ea02078\n\t", "INSPVAXA,USB3,0,47.5,FINESTEERING,2107,282902.100,02000000,471d,15824;INS_ALIGNMENT_COMPLETE,INS_RTKFIXED,37.37089489898,126.72382363217,9.0942,22.3000,0.2058,-0.2206,-0.0113,0.048071178,-2.299077036,298.376589904,0.4428,0.2943,0.5540,0.1136,0.0924,0.0773,0.0981,0.1029,4.8877,0f000001,0*27878755\n\t", "INSPVAXA,USB3,0,47.5,FINESTEERING,2107,282902.600,02000000,471d,15824;INS_ALIGNMENT_COMPLETE,INS_RTKFIXED,37.37089561933,126.72382228336,9.0897,22.3000,0.2051,-0.2120,-0.0118,0.043026481,-2.382631281,298.375025440,0.4428,0.2943,0.5540,0.1136,0.0924,0.0773,0.0981,0.1029,4.8877,0f000001,0*7b155814\n\t", "INSPVAXA,USB3,0,50.5,FINESTEERING,2107,282903.100,02000000,471d,15824;INS_ALIGNMENT_COMPLETE,INS_RTKFIXED,37.37089633791,126.72382096695,9.0851,22.3000,0.2033,-0.2166,-0.0158,0.077766570,-2.447937912,298.353889057,0.4425,0.2944,0.5540,0.1136,0.0924,0.0773,0.0981,0.1029,4.8888,0f000001,0*d3856956\n\t", "INSPVAXA,USB3,0,50.5,FINESTEERING,2107,282903.600,02000000,471d,15824;INS_ALIGNMENT_COMPLETE,INS_RTKFIXED,37.37089705589,126.72381965369,9.0797,22.3000,0.2030,-0.2155,-0.0169,0.162662561,-2.490332346,298.323964728,0.4425,0.2944,0.5540,0.1136,0.0924,0.0773,0.0981,0.1029,4.8888,0f000001,0*903bf558\n\t", "INSPVAXA,USB3,0,48.5,FINESTEERING,2107,282904.100,02000000,471d,15824;INS_ALIGNMENT_COMPLETE,INS_RTKFIXED,37.37089779647,126.72381832272,9.0739,22.3000,0.1899,-0.2136,-0.0154,0.294805164,-2.652846307,298.299564354,0.4429,0.2945,0.5544,0.1137,0.0925,0.0774,0.0981,0.1030,4.8900,0f000001,0*1aba8cff\n\t", "INSPVAXA,USB3,0,42.5,FINESTEERING,2107,282905.100,02000000,471d,15824;INS_ALIGNMENT_COMPLETE,INS_RTKFIXED,37.37089924281,126.72381565825,9.0621,22.3000,0.2032,-0.2264,-0.0151,0.296199790,-2.500120429,298.405278935,0.4415,0.2943,0.5538,0.1135,0.0924,0.0773,0.0981,0.1029,4.8913,0f000001,0*c27d96a4\n\t", "INSPVAXA,USB3,0,42.5,FINESTEERING,2107,282905.600,02000000,471d,15824;INS_ALIGNMENT_COMPLETE,INS_RTKFIXED,37.37089993990,126.72381433650,9.0561,22.3000,0.1965,-0.2206,-0.0194,0.175024687,-2.429152117,298.413626254,0.4415,0.2943,0.5538,0.1135,0.0924,0.0773,0.0981,0.1029,4.8913,0f000001,0*60204f40\n\t", "INSPVAXA,USB3,0,50.0,FINESTEERING,2107,282906.100,02000000,471d,15824;INS_ALIGNMENT_COMPLETE,INS_RTKFIXED,37.37090067392,126.72381297631,9.0488,22.3000,0.1869,-0.2231,-0.0278,0.198226586,-2.470510374,298.476445158,0.4408,0.2943,0.5536,0.1134,0.0924,0.0773,0.0981,0.1029,4.8926,0f000001,0*c8d31ab7\n\t", "INSPVAXA,USB3,0,50.0,FINESTEERING,2107,282906.600,02000000,471d,15824;INS_ALIGNMENT_COMPLETE,INS_RTKFIXED,37.37090140156,126.72381162044,9.0410,22.3000,0.1900,-0.2268,-0.0250,0.233406583,-2.464396388,298.527307451,0.4408,0.2943,0.5536,0.1134,0.0924,0.0773,0.0981,0.1029,4.8926,0f000001,0*6dbb954e\n\t", "INSPVAXA,USB3,0,47.5,FINESTEERING,2107,282907.100,02000000,471d,15824;INS_ALIGNMENT_COMPLETE,INS_RTKFIXED,37.37090211288,126.72381031698,9.0345,22.3000,0.1914,-0.2193,-0.0163,0.234265658,-2.429917565,298.557656131,0.4407,0.2944,0.5534,0.1135,0.0925,0.0773,0.0981,0.1029,4.8940,0f000001,0*98d66c71\n\t", "INSPVAXA,USB3,0,47.5,FINESTEERING,2107,282907.600,02000000,471d,15824;INS_ALIGNMENT_COMPLETE,INS_RTKFIXED,37.37090284953,126.72380892748,9.0281,22.3000,0.1780,-0.2041,-0.0150,0.112459051,-2.561733911,298.657756217,0.4407,0.2944,0.5534,0.1135,0.0925,0.0773,0.0981,0.1029,4.8940,0f000001,0*46e93b24\n\t", "INSPVAXA,USB3,0,47.5,FINESTEERING,2107,282908.100,02000000,471d,15824;INS_ALIGNMENT_COMPLETE,INS_RTKFIXED,37.37090357557,126.72380757332,9.0217,22.3000,0.2057,-0.2321,-0.0149,0.061524953,-2.489801509,298.773706778,0.4409,0.2944,0.5534,0.1134,0.0925,0.0773,0.0981,0.1029,4.8951,0f000001,0*737dd3e1\n\t", "INSPVAXA,USB3,0,42.5,FINESTEERING,2107,282908.600,02000000,471d,15824;INS_ALIGNMENT_COMPLETE,INS_RTKFIXED,37.37090428415,126.72380622581,9.0150,22.3000,0.1993,-0.2229,-0.0194,0.018544103,-2.459857959,298.845685977,0.4409,0.2944,0.5534,0.1134,0.0925,0.0773,0.0981,0.1029,4.8951,0f000001,0*f932705e\n\t", "INSPVAXA,USB3,0,45.5,FINESTEERING,2107,282909.100,02000000,471d,15824;INS_ALIGNMENT_COMPLETE,INS_RTKFIXED,37.37090502254,126.72380483216,9.0074,22.3000,0.1877,-0.2104,-0.0206,-0.090329657,
